vi "Write Data.vi"(8 "error in (no error)":errorcluster, 9 "Publication Time":timestamp, 10 "Value":variant, 11 "TerminalEnabledStateBinding In":refnum<class "TerminalEnabledStateBinding.lvclass">) -> (0 "error out":errorcluster, 3 "TerminalEnabledStateBinding Out":refnum<class "TerminalEnabledStateBinding.lvclass">)   [LabVIEW 2017, in "Transport.lvlib" / "TerminalEnabledStateBinding.lvclass"]
doc: "<License>\nCopyright © 2017 Composed Systems, LLC | All rights reserved\nwww.composed.io\n\nAuthor: Ethan Stern <ethan.stern@composed.io>\n\nThis software is provided \"AS IS\" WITHOUT WARRANTIES, either express or implied, AND IS FOR EDUCATIONAL PURPOSES ONLY.\n</License>"
uses:
  TerminalEnabledStateBinding.lvclass
  TerminalEnabledStateBinding.lvclass/TerminalEnabledStateBinding.ctl
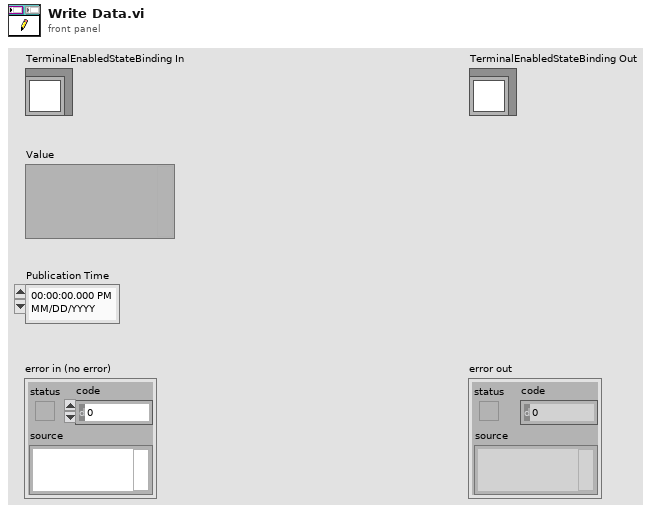
[diagram p1: front panel]
types:
  T1 = enum8{"Enabled", "Disabled", "Disabled and Grayed Out"}
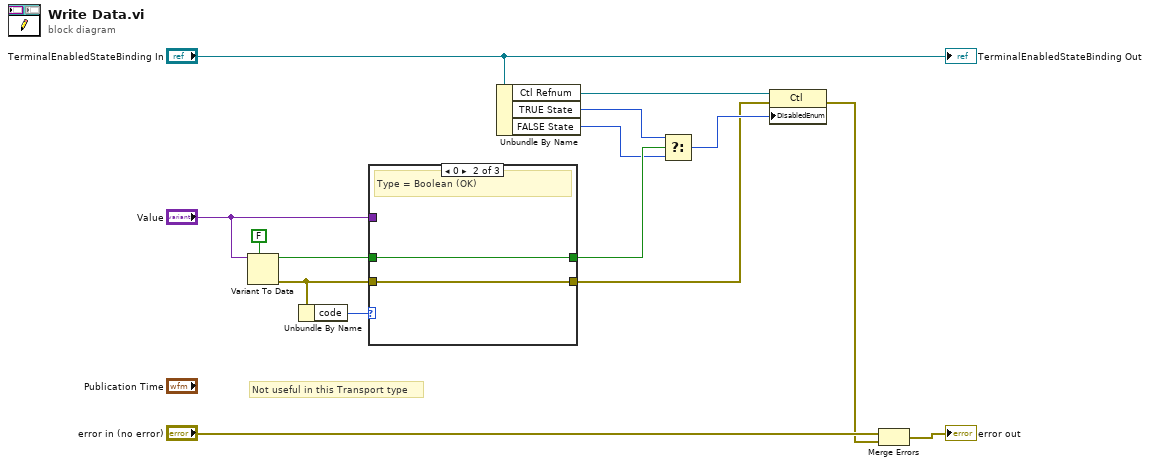
[diagram p0: block diagram]
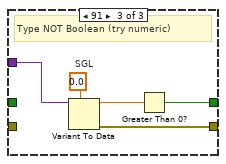
[diagram p3: hidden frame]
diagram:
  # "Not useful in this Transport type"
  n1 = Variant To Data(type=FALSE, Variant="Value") -> (data=w7:bool, error out=w6:errorcluster)  [unwired: 1 in]
  n2 = Unbundle By Name(w6) -> ("code"=w8:i32)
  n3 = case shown="0" w8 {
    tunnel: w7 -> [w17 w19 _]
    tunnel: [w17 w19 w22] -> w2
    tunnel: "Value" -> [_ _ w21]
    tunnel: [w16 w18 w20] -> w5
    tunnel: w6 -> [w16 w18 _]
    frame Default {
      # "A more serious (unexpected) error"
    }
    frame 0 {
      # "Type = Boolean (OK)"
    }
    frame 91 {
      w24 = sgl 0.0  # SGL
      # "Type NOT Boolean (try numeric)"
      n4 = Variant To Data(type=w24, Variant=w21) -> (data=w23:sgl, error out=w20:errorcluster)  [unwired: 1 in]
      n5 = Greater Than 0?(x=w23) -> (x > 0?=w22:bool)
    }
  }
  n6 = Unbundle By Name("TerminalEnabledStateBinding In") -> ("Ctl Refnum"=w13:refnum<vi>, "TRUE State"=w3:T1, "FALSE State"=w1:T1)
  n7 = Select(t=w3, s=w2, f=w1) -> (s? t:f=w9:T1)
  n8 = property class="Ctl"(reference=w13, error in=w5, "DisabledEnum"=w9) -> (error out=w11:errorcluster)  [unwired: 1 out]
  n9 = Merge Errors("error in (no error)", w11) -> (→"error out":errorcluster)
  "TerminalEnabledStateBinding Out" <- "TerminalEnabledStateBinding In"
